vi "HFRR ADV v01.vi"() -> ()   [LabVIEW 2025] (continued)
          selector: w1771 -> [_ w1776]
          frame False {
          }
          frame True {
            n1472 = Not(x=w1776) -> (.not. x?=w1775:bool)
            n1473 = local write "CAMERA ROI MIN TEMP"(w1775) -> ()
            n1474 = call "IMAGE ANALYSIS.vi"("Enum"=POST_ANALYSIS_ENUM."MINIMIZE UI") -> ()  [unwired: 9 in, 2 out]
          }
        }
        n1475 = local write "CAMERA ROI MAX TEMP"(TRUE ("CAMERA ROI MIN TEMP")) -> ()
      }
      frame "Advance" {
        n1476 = local read "LIVE FEED MIN TEMP"() -> (w1782:bool)
        n1477 = local write "LIVE FEED MAX TEMP"(TRUE ("LIVE FEED MAX TEMP")) -> ()
        n1478 = local read "CAMERA ROI MIN TEMP"() -> (w1780:bool)
        n1479 = case shown="True" w1782 {
          selector: w1782 -> [_ w1789]
          frame False {
          }
          frame True {
            n1480 = Not(x=w1789) -> (.not. x?=w1788:bool)
            n1481 = local write "LIVE FEED MIN TEMP"(w1788) -> ()
            n1482 = call "CAMERA LIVE FEED FGV.vi"("Enum - Menu"=CAMERA_LIVE_FEED_ENUM."CAMERA MINIMIZE") -> ()  [unwired: 9 in, 2 out]
          }
        }
        n1483 = local write "CAMERA ROI MAX TEMP"(TRUE ("CAMERA ROI MAX TEMP")) -> ()
        n1484 = case shown="True" w1780 {
          selector: w1780 -> [_ w1786]
          frame False {
          }
          frame True {
            n1485 = Not(x=w1786) -> (.not. x?=w1785:bool)
            n1486 = local write "CAMERA ROI MIN TEMP"(w1785) -> ()
            n1487 = call "IMAGE ANALYSIS.vi"("Enum"=POST_ANALYSIS_ENUM."MINIMIZE UI") -> ()  [unwired: 9 in, 2 out]
          }
        }
      }
      frame "Mooha" {
        n1488 = local read "LIVE FEED MIN TEMP"() -> (w1792:bool)
        n1489 = local write "LIVE FEED MAX TEMP"(TRUE ("LIVE FEED MAX TEMP")) -> ()
        n1490 = local read "CAMERA ROI MIN TEMP"() -> (w1790:bool)
        n1491 = case shown="True" w1792 {
          selector: w1792 -> [_ w1799]
          frame False {
          }
          frame True {
            n1492 = Not(x=w1799) -> (.not. x?=w1798:bool)
            n1493 = local write "LIVE FEED MIN TEMP"(w1798) -> ()
            n1494 = call "CAMERA LIVE FEED FGV.vi"("Enum - Menu"=CAMERA_LIVE_FEED_ENUM."CAMERA MINIMIZE") -> ()  [unwired: 9 in, 2 out]
          }
        }
        n1495 = local write "CAMERA ROI MAX TEMP"(TRUE ("CAMERA ROI MAX TEMP")) -> ()
        n1496 = case shown="True" w1790 {
          selector: w1790 -> [_ w1796]
          frame False {
          }
          frame True {
            n1497 = Not(x=w1796) -> (.not. x?=w1795:bool)
            n1498 = local write "CAMERA ROI MIN TEMP"(w1795) -> ()
            n1499 = call "IMAGE ANALYSIS.vi"("Enum"=POST_ANALYSIS_ENUM."MINIMIZE UI") -> ()  [unwired: 9 in, 2 out]
          }
        }
      }
    }
    n1500 = local read "Auto Start Test"() -> (w1537:bool)
    n1501 = case shown="True" "sign in temp" {
      frame False {
      }
      frame True {
        w1572 = 1 ("y")
        n1502 = local read "USERNAME"() -> (w1578:string)
        n1503 = local read "USER ID"() -> (w1575:string)
        n1504 = call <vilib>:"Trim Whitespace.vi"("string"=w1578) -> ("trimmed string"=w1577:string)  [unwired: 1 in]
        n1505 = call <vilib>:"Trim Whitespace.vi"("string"=w1575) -> ("trimmed string"=w1576:string)  [unwired: 1 in]
        n1506 = String Length(string=w1577) -> (length=w1574:i32)
        n1507 = String Length(string=w1576) -> (length=w1573:i32)
        n1508 = Greater?(x=w1574, y=w1572) -> (0:w1571:bool)
        n1509 = Greater?(x=w1573, y=w1572) -> (0:w1570:bool)
        n1510 = And(x=w1571, y=w1570) -> (x .and. y?=w1569:bool)
        n1511 = case shown="True" w1569 {
          frame False {
            n1512 = property on="Sign In" class="Bool (strict)"("DisabledEnum"=T19."Disabled" ("Disabled")) -> ()  [unwired: 2 in, 2 out]
          }
          frame True {
            n1513 = property on="Sign In" class="Bool (strict)"("DisabledEnum"=T19."Enabled" ("Disabled")) -> ()  [unwired: 2 in, 2 out]
          }
        }
      }
    }
    n1514 = local read "Air Temperature"() -> (w1554:bool)
    n1515 = local read "Coefficient Of Friction"() -> (w1555:bool)
    n1516 = case shown="False" w1537 {
      frame False {
        n1517 = local read "Auto stop temp"() -> (w1566:bool)
        n1518 = case shown="True" w1566 {
          frame False {
          }
          frame True {
            n1519 = local write "Auto Start Temp"(FALSE ("Auto Start Temp")) -> ()
          }
        }
      }
      frame True {
        "Auto stop temp" <- TRUE ("Auto stop temp")
      }
    }
    n1520 = local read "Humidity 3"() -> (w1553:bool)
    n1521 = case shown="\"HOME\"" w1563 {
      frame "HOME" {
        n1522 = local write "main tab sub"(enum32{"Page 1", "Page 2"}."Page 1" ("main tab sub")) -> ()
      }
      frame Default {
        n1523 = local write "main tab sub"(enum32{"Page 1", "Page 2"}."Page 2" ("main tab sub")) -> ()
      }
    }
    n1524 = case shown="True" w1562 {
      selector: w1562 -> [_ w1914]
      frame False {
      }
      frame True {
        n1525 = Not(x=w1914) -> (.not. x?=w1913:bool)
        n1526 = local write "Sign In"(w1913) -> ()
        n1527 = local write "Main Dashboard Buttons"(T25."Test Setup" ("Main Dashboard Buttons")) -> ()
      }
    }
    n1528 = case shown="\"Numeric Display\", Default" "Num/Graph" {
      frame "Numeric Display", Default {
        n1529 = property on="Single/Multiple" class="RadioBtnsControl (strict)"("Visible"=FALSE) -> ()  [unwired: 2 in, 2 out]
        n1530 = property on="Single - Graph" class="Ring (strict)"("Visible"=FALSE) -> ()  [unwired: 2 in, 2 out]
        n1531 = local write "Main Tab Display"(T6."Dashboard 1" ("Main Tab Display")) -> ()
      }
      frame "Graph Display" {
        n1532 = property on="Single/Multiple" class="RadioBtnsControl (strict)"("Visible"=TRUE) -> ()  [unwired: 2 in, 2 out]
        n1533 = case shown="\"Multiple\"" "Single/Multiple" {
          frame "Single ", Default {
            n1534 = property on="Single - Graph" class="Ring (strict)"("Visible"=TRUE) -> ()  [unwired: 2 in, 2 out]
            n1535 = local write "Main Tab Display"(T6."Dashboard 3" ("Main Tab Display")) -> ()
          }
          frame "Multiple" {
            n1536 = property on="Single - Graph" class="Ring (strict)"("Visible"=FALSE) -> ()  [unwired: 2 in, 2 out]
            n1537 = local write "Main Tab Display"(T6."Dashboard 2" ("Main Tab Display")) -> ()
          }
        }
      }
    }
    n1538 = local read "Stroke"() -> (w1552:bool)
    n1539 = local read "USERNAME"() -> (w1557:string)
    n1540 = case shown="True" w1555 {
      selector: w1555 -> [_ w1839]
      frame False {
      }
      frame True {
        n1541 = Not(x=w1839) -> (.not. x?=w1838:bool)
        n1542 = local write "Coefficient Of Friction"(w1838) -> ()
        n1543 = local write "Tab Control 2"(T8."Coefficient Of Friction" ("Tab Control 2")) -> ()
      }
    }
    n1544 = case shown="True" w1554 {
      selector: w1554 -> [_ w1836]
      frame False {
      }
      frame True {
        n1545 = Not(x=w1836) -> (.not. x?=w1834:bool)
        n1546 = local write "Air Temperature"(w1834) -> ()
        n1547 = local write "Tab Control 2"(T8."Air Temperature" ("Tab Control 2")) -> ()
      }
    }
    n1548 = case shown="True" w1552 {
      selector: w1552 -> [_ w1830]
      frame False {
      }
      frame True {
        n1549 = Not(x=w1830) -> (.not. x?=w1828:bool)
        n1550 = local write "Stroke"(w1828) -> ()
        n1551 = local write "Tab Control 2"(T8."Stroke" ("Tab Control 2")) -> ()
      }
    }
    n1552 = local write "tested by"(w1557) -> ()
    n1553 = case shown="True" w1553 {
      selector: w1553 -> [_ w1833]
      frame False {
      }
      frame True {
        n1554 = Not(x=w1833) -> (.not. x?=w1831:bool)
        n1555 = local write "Humidity 3"(w1831) -> ()
        n1556 = local write "Tab Control 2"(T8."Humidity" ("Tab Control 2")) -> ()
      }
    }
    n1557 = case shown="\"Calibration\"" "Main Dashboard Buttons" {
      tunnel: [T4."HOME" ("Main Tab") T4."Test Setup" ("Main Tab") T4."Acquire" ("Main Tab") T4."Adv Scar" ("Main Tab") T4."Adv Scar Report" ("Main Tab") T4."Compare Files" ("Main Tab") T4."Calibration" ("Main Tab") T4."About" ("Main Tab") T4."Advance" ("Main Tab")] -> w1536
      frame "Home", Default {
      }
      frame "Test Setup" {
      }
      frame "Dashboard" {
      }
      frame "Imaging" {
      }
      frame "Report" {
      }
      frame "Analysis" {
      }
      frame "Calibration" {
      }
      frame "About" {
      }
      frame "Advance" {
      }
    }
    n1558 = Wait (ms)(milliseconds to wait=u32 100) -> ()  [unwired: 1 out]
    n1559 = local read "Main Tab Display"() -> (w1556:T6)
    n1560 = local write "Main Tab"(w1536) -> ()
    n1561 = case shown="\"Dashboard 3\"" w1556 {
      frame "Dashboard 1", Default {
        n1562 = property on="Reset Graph" class="Bool (strict)"("Visible"=FALSE) -> ()  [unwired: 2 in, 2 out]
      }
      frame "Dashboard 2" {
        n1563 = property on="Reset Graph" class="Bool (strict)"("Visible"=TRUE) -> ()  [unwired: 2 in, 2 out]
      }
      frame "Dashboard 3" {
        n1564 = property on="Reset Graph" class="Bool (strict)"("Visible"=TRUE) -> ()  [unwired: 2 in, 2 out]
      }
    }
    n1565 = local read "SCAR MEASURMENT"() -> (w1544:enum32{"Auto Scar", "Manual Scar"})
    n1566 = local read "Humidity"() -> (w1558:bool)
    n1567 = local read "Cap Live Image"() -> (w1541:bool)
    n1568 = local read "Sample Temperature"() -> (w1551:bool)
    n1569 = local read "Air Temp vs Humidity"() -> (w1549:bool)
    n1570 = local read "Frequency"() -> (w1550:bool)
    n1571 = case shown="False" w1558 {
      frame False {
        n1572 = local write "Humidity On Command"(TRUE ("Humidity On Command")) -> ()
        n1573 = case shown="True" "Humidity Off Command" {
          selector: "Humidity Off Command" -> [_ w1846]
          frame False {
          }
          frame True {
            n1574 = stacked-sequence {
              frame #0 {
                n1575 = local read "WriteHumidity"() -> (w1848:string[])
                n1576 = Insert Into Array(array=w1848, new element="R;1" ("new element/subarray")) -> (w1847:string[])  [unwired: 1 in]
                n1577 = local write "WriteHumidity"(w1847) -> ()
              }
              frame #1 {
                n1578 = Wait (ms)(milliseconds to wait=u32 500) -> ()  [unwired: 1 out]
              }
              frame #2 {
                n1579 = local read "WriteHumidity"() -> (w1852:string[])
                n1580 = local read "EVENT LOG"() -> (w1856:string)
                n1581 = call "Event Log.vi"("Content"="Humidity Control Off" ("string"), "EVENT LOG"=w1856) -> ("EVENT LOG"=w1857:string)  [unwired: 8 in, 1 out]
                n1582 = local write "EVENT LOG"(w1857) -> ()
                n1583 = Insert Into Array(array=w1852, new element="R;1" ("new element/subarray")) -> (w1853:string[])  [unwired: 1 in]
                n1584 = local write "WriteHumidity"(w1853) -> ()
                n1585 = local write "Humidity 2"(TRUE ("Humidity")) -> ()
              }
            }
            n1586 = Not(x=w1846) -> (.not. x?=w1845:bool)
            n1587 = local write "Humidity Off Command"(w1845) -> ()
          }
        }
      }
      frame True {
        n1588 = local write "Humidity Off Command"(TRUE ("Humidity Off Command")) -> ()
        n1589 = case shown="False" "Humidity On Command" {
          selector: "Humidity On Command" -> [_ w1861]
          frame False {
          }
          frame True {
            n1590 = stacked-sequence {
              frame #0 {
                n1591 = local read "Set Rh"() -> (w1867:dbl)
                n1592 = local read "WriteHumidity"() -> (w1863:string[])
                n1593 = Number To Fractional String(number=w1867, precision (6)=i16 2) -> (F-format string=w1868:string)  [unwired: 2 in]
                n1594 = Concatenate Strings("M;" ("new element/subarray"), w1868) -> (w1866:string)
                n1595 = Insert Into Array(array=w1863, new element=w1866) -> (w1862:string[])  [unwired: 1 in]
                n1596 = local write "WriteHumidity"(w1862) -> ()
              }
              frame #1 {
                n1597 = Wait (ms)(milliseconds to wait=u32 500) -> ()  [unwired: 1 out]
              }
              frame #2 {
                n1598 = local read "WriteHumidity"() -> (w1871:string[])
                n1599 = local read "Set Rh"() -> (w1875:dbl)
                n1600 = Number To Fractional String(number=w1875, precision (6)=i16 2) -> (F-format string=w1876:string)  [unwired: 2 in]
                n1601 = Concatenate Strings("M;" ("new element/subarray"), w1876) -> (w1874:string)
                n1602 = Insert Into Array(array=w1871, new element=w1874) -> (w1870:string[])  [unwired: 1 in]
                n1603 = local write "WriteHumidity"(w1870) -> ()
              }
              frame #3 {
                n1604 = Wait (ms)(milliseconds to wait=u32 500) -> ()  [unwired: 1 out]
              }
              frame #4 {
                (unwired) "% RH" ("string")
                (unwired) i16 2 ("precision (6)")
                (unwired) "M;" ("new element/subarray")
                n1605 = local read "Set Rh"() -> (w1885:dbl)
                n1606 = local read "WriteHumidity"() -> (w1878:string[])
                n1607 = Number To Fractional String(number=w1885, precision (6)=i16 2) -> (F-format string=w1882:string)  [unwired: 2 in]
                n1608 = Concatenate Strings("M;" ("new element/subarray"), w1882) -> (w1886:string)
                n1609 = Concatenate Strings("Humidity Set to : " ("string"), w1882, "% RH" ("string")) -> (w1880:string)
                n1610 = Insert Into Array(array=w1878, new element=w1886) -> (w1879:string[])  [unwired: 1 in]
                n1611 = disable-structure shown="Enabled" {
                  frame Enabled {
                    n1612 = local read "EVENT LOG"() -> (w1889:string)
                    n1613 = call "Event Log.vi"("Content"="Humidity Control On", "EVENT LOG"=w1889) -> ("EVENT LOG"=w1890:string)  [unwired: 8 in, 1 out]
                    n1614 = local write "EVENT LOG"(w1890) -> ()
                  }
                  frame Disabled {
                  }
                }
                n1615 = disable-structure shown="Enabled" {
                  disable-tunnel: w1880 -> [_ _]
                  frame Enabled {
                    n1616 = local read "EVENT LOG"() -> (w1892:string)
                    n1617 = call "Event Log.vi"("Content"="Humidity Control On", "EVENT LOG"=w1892) -> ("EVENT LOG"=w1893:string)  [unwired: 8 in, 1 out]
                    n1618 = local write "EVENT LOG"(w1893) -> ()
                  }
                  frame Disabled {
                  }
                }
                n1619 = local write "WriteHumidity"(w1879) -> ()
              }
            }
            n1620 = Not(x=w1861) -> (.not. x?=w1860:bool)
            n1621 = local write "Humidity On Command"(w1860) -> ()
          }
        }
      }
    }
    n1622 = Equal?(x=w1544, y=enum32{"Auto Scar", "Manual Scar"}."Auto Scar" ("SCAR MEASURMENT")) -> (x = y?=w1540:bool)
    n1623 = local read "TEST STANDARD"() -> (w1547:T5)
    n1624 = And(x=w1541, y=w1540) -> (x .and. y?=w1542:bool)
    n1625 = case shown="True" w1542 {
      selector: w1542 -> [_ w1645]
      tunnel: errorcluster {"status"=FALSE, "code"=0, "source"=""} ("error in (no error) 3") -> [_ w1646]
      frame False {
      }
      frame True {
        n1626 = stacked-sequence {
          tunnel: w1646 -> [_ _ _ _ _ _ _ w1694]
          tunnel: w1645 -> [_ _ _ _ _ w1675 _ _]
          frame #0 {
            n1627 = call "CAMERA LIVE FEED FGV.vi"("Enum - Menu"=CAMERA_LIVE_FEED_ENUM."CAMERA MINIMIZE") -> ()  [unwired: 9 in, 2 out]
          }
          frame #1 {
            n1628 = property on="Auto Scar Check  2" class="Clust (strict)"("Visible"=TRUE) -> ()  [unwired: 2 in, 2 out]
          }
          frame #2 {
            n1629 = String To Path(string="C:\\LAB-IQ\\Image Calibrate v01.dcf") -> (path=w1651:path)
            n1630 = Open/Create/Replace File ("Open File")(file path (use dialog)=w1651) -> (refnum out=w1652:refnum<file>)  [unwired: 5 in, 2 out]
            n1631 = for {
              N: 4 -> [_]
              tunnel: w1652 -> [w1658]
              i -> [w1654]
              n1632 = Read from Text File ("Read File")(file (use dialog)=w1658) -> (text=w1659:string)  [unwired: 3 in, 3 out]
              n1633 = String Subset(string=w1659, offset (0)=6, length (rest)=10 ("length (rest)")) -> (substring=w1655:string)
              n1634 = Fract/Exp String To Number(string=w1655) -> (number=w1653:dbl)  [unwired: 3 in, 1 out]
              n1635 = case shown="0" w1654 {
                tunnel: w1653 -> [w1660 w1661 _ w1662 _]
                frame 0 {
                  "5x Gain" <- w1660
                }
                frame 1 {
                  "10x Gain" <- w1661
                }
                frame 2 {
                }
                frame 3 {
                  "100x gain" <- w1662
                }
                frame 4, Default {
                }
              }
            }
          }
          frame #3 {
            n1636 = local read "FILE 3"() -> (w1668:string)
            n1637 = call <vilib>:"Trim Whitespace.vi"("string"="C:\\LAB-IQ\\images\\") -> ("trimmed string"=w1670:string)  [unwired: 1 in]
            n1638 = String To Path(string=w1670) -> (path=w1669:path)
            n1639 = Concatenate Strings(w1668, ".png" ("string")) -> (w1667:string)
            n1640 = Build Path(base path=w1669, name or relative path=w1667) -> (appended path=w1665:path)
            "Image path" <- w1665
            n1641 = Path To String(path=w1665) -> (string=w1664:string)
            n1642 = call "CAMERA LIVE FEED FGV.vi"("Enum - Menu"=CAMERA_LIVE_FEED_ENUM."CAMERA SAVE", "Image Path"=w1664) -> ()  [unwired: 8 in, 2 out]
          }
          frame #4 {
            n1643 = One Button Dialog(message="Image saved successfully") -> ()  [unwired: 1 in, 1 out]
          }
          frame #5 {
            n1644 = local read "TEST STANDARD"() -> (w1674:T5)
            n1645 = local read "Magnification len live scar"() -> (w1686:string)
            n1646 = Not(x=w1675) -> (.not. x?=w1676:bool)
            n1647 = local write "Cap Live Image"(w1676) -> ()
            n1648 = case shown="\"ISO 12156\"" w1674 {
              tunnel: ["ASTM D6079" "ISO 12156"] -> w1673
              frame "ASTM D6079", Default {
              }
              frame "ISO 12156" {
              }
            }
            n1649 = case shown="\"5x\", Default" w1686 {
              tunnel: [w1689 w1690] -> w1685
              frame "5x", Default {
                n1650 = local read "5x Gain"() -> (w1689:dbl)
              }
              frame "10x" {
                # "5x"
                n1651 = local read "10x Gain"() -> (w1690:dbl)
              }
            }
            n1652 = local read "Image path"() -> (w1684:path)
            n1653 = local read "FILE 3"() -> (w1677:string)
            n1654 = call "EDGE DETCTION.vi"("GAIN VALUE"=w1685, "Image Path"=w1684) -> ("error out"=w1683:errorcluster, "return value"=w1682:cluster{string, string, dbl, dbl, dbl})  [unwired: 8 in]
            n1655 = Bundle By Name(cluster=T26 {"File Name"="", "Test Method"="", "Operator"="", "Fuel Description"="", "Date and time"=""} ("Main Ref"), "File Name"=w1677, "Test Method"=w1673) -> (w1678:T26)
            n1656 = call "duf file read.vi"("error in (no error)"=w1683, "Main Ref"=w1678) -> ("error out"=w1681:errorcluster, "Main Ref 2"=w1679:T26)  [unwired: 8 in]
            n1657 = call "EDGE DETECTION REPORT.vi"("error in (no error)"=w1681, "return value 2"=w1682, "Main Ref"=w1679) -> ()  [unwired: 8 in, 1 out]
          }
          frame #6 {
            n1658 = property on="Auto Scar Check  2" class="Clust (strict)"("Visible"=FALSE) -> ()  [unwired: 2 in, 2 out]
          }
          frame #7 {
            n1659 = call "CAMERA LIVE FEED FGV.vi"("Enum - Menu"=CAMERA_LIVE_FEED_ENUM."CAMERA MINIMIZE", "error in (no error)"=w1694) -> ()  [unwired: 8 in, 2 out]
            n1660 = local write "Main Dashboard Buttons"(T1."Home" ("Main Dashboard Buttons")) -> ()
            n1661 = local write "Main Tab"(T4."HOME" ("Main Tab")) -> ()
          }
        }
      }
    }
    n1662 = local read "Heater Button"() -> (w1548:bool)
    n1663 = case shown="True" w1550 {
      selector: w1550 -> [_ w1824]
      frame False {
      }
      frame True {
        n1664 = Not(x=w1824) -> (.not. x?=w1822:bool)
        n1665 = local write "Frequency"(w1822) -> ()
        n1666 = local write "Tab Control 2"(T8."Frequency" ("Tab Control 2")) -> ()
      }
    }
    n1667 = case shown="True" w1549 {
      selector: w1549 -> [_ w1821]
      frame False {
      }
      frame True {
        n1668 = Not(x=w1821) -> (.not. x?=w1819:bool)
        n1669 = local write "Air Temp vs Humidity"(w1819) -> ()
        n1670 = local write "Tab Control 2"(T8."Air Temp vs Rh" ("Tab Control 2")) -> ()
      }
    }
    n1671 = case shown="True" w1551 {
      selector: w1551 -> [_ w1827]
      frame False {
      }
      frame True {
        n1672 = Not(x=w1827) -> (.not. x?=w1825:bool)
        n1673 = local write "Sample Temperature"(w1825) -> ()
        n1674 = local write "Tab Control 2"(T8."Sample Temperature" ("Tab Control 2")) -> ()
      }
    }
    n1675 = case shown="\"Custom\"" w1547 {
      frame "ASTM D6079", Default {
        w1800 = "ASTM D6079 TEST CONDITIONS" ("Standard 2")
        n1676 = local write "Standard 2"(w1800) -> ()
        n1677 = local write "Standard"(w1800) -> ()
      }
      frame "ISO 12156" {
        w1801 = "ISO 12156 TEST CONDITIONS" ("Standard 2")
        n1678 = local write "Standard 2"(w1801) -> ()
        n1679 = local write "Standard"(w1801) -> ()
      }
      frame "CEC F-096-A-06" {
        w1802 = "CEC F-096-A-06 TEST CONDITIONS" ("Standard 2")
        n1680 = local write "Standard 2"(w1802) -> ()
        n1681 = local write "Standard"(w1802) -> ()
      }
      frame "Custom" {
        w1803 = "CUSTOM TEST CONDITIONS" ("Standard 2")
        n1682 = local write "Standard 2"(w1803) -> ()
        n1683 = local write "Standard"(w1803) -> ()
      }
    }
    n1684 = case shown="True" w1548 {
      frame False {
        n1685 = local write "Temperature On Command"(TRUE ("Temperature On Command")) -> ()
        n1686 = case shown="True" "Temperature Off Command" {
          selector: "Temperature Off Command" -> [_ w1807]
          frame False {
          }
          frame True {
            n1687 = Not(x=w1807) -> (.not. x?=w1806:bool)
            n1688 = local read "EVENT LOG"() -> (w1810:string)
            n1689 = local write "Temperature Off Command"(w1806) -> ()
            n1690 = call "Event Log.vi"("Content"="Heater Off", "EVENT LOG"=w1810) -> ("EVENT LOG"=w1809:string)  [unwired: 8 in, 1 out]
            n1691 = local write "EVENT LOG"(w1809) -> ()
          }
        }
      }
      frame True {
        n1692 = local write "Temperature Off Command"(TRUE ("Temperature Off Command")) -> ()
        n1693 = case shown="True" "Temperature On Command" {
          selector: "Temperature On Command" -> [_ w1814]
          frame False {
          }
          frame True {
            n1694 = Not(x=w1814) -> (.not. x?=w1813:bool)
            n1695 = local write "Temperature On Command"(w1813) -> ()
            n1696 = disable-structure shown="Enabled" {
              disable-tunnel: "Heater On" -> [w1816 _]
              frame Enabled {
                n1697 = local read "EVENT LOG"() -> (w1817:string)
                n1698 = call "Event Log.vi"("Content"=w1816, "EVENT LOG"=w1817) -> ("EVENT LOG"=w1818:string)  [unwired: 8 in, 1 out]
                n1699 = local write "EVENT LOG"(w1818) -> ()
              }
              frame Disabled {
              }
            }
          }
        }
      }
    }
    n1700 = local read "Main Tab"() -> (w1539:T4)
    n1701 = case shown="\"About\"" w1539 {
      frame "HOME", Default {
        w1581 = T19."Enabled" ("Disabled")
        n1702 = local read "Service Password enable"() -> (w1583:bool)
        n1703 = property on="Imaging" class="Bool (strict)"("DisabledEnum"=w1581) -> ()  [unwired: 2 in, 2 out]
        n1704 = property on="Dashboard" class="Bool (strict)"("DisabledEnum"=w1581) -> ()  [unwired: 2 in, 2 out]
        n1705 = property on="Test Setup" class="Bool (strict)"("DisabledEnum"=w1581) -> ()  [unwired: 2 in, 2 out]
        n1706 = property on="Analysis" class="Bool (strict)"("DisabledEnum"=w1581) -> ()  [unwired: 2 in, 2 out]
        n1707 = property on="Home" class="Bool (strict)"("DisabledEnum"=w1581) -> ()  [unwired: 2 in, 2 out]
        n1708 = property on="Report" class="Bool (strict)"("DisabledEnum"=w1581) -> ()  [unwired: 2 in, 2 out]
        n1709 = property on="Main Dashboard Buttons" class="RadioBtnsControl (strict)"("DisabledEnum"=w1581) -> ()  [unwired: 2 in, 2 out]
        n1710 = property on="Calibration" class="Bool (strict)"("DisabledEnum"=w1581) -> ()  [unwired: 2 in, 2 out]
        n1711 = case shown="True" w1583 {
          tunnel: [T19."Disabled" ("Disabled") T19."Enabled" ("Disabled")] -> w1582
          frame False {
          }
          frame True {
          }
        }
        n1712 = property on="About" class="Bool (strict)"("DisabledEnum"=w1582) -> ()  [unwired: 2 in, 2 out]
      }
      frame "Test Setup" {
        w1588 = T19."Enabled" ("Disabled")
        n1713 = local read "Service Password enable"() -> (w1587:bool)
        n1714 = property on="Dashboard" class="Bool (strict)"("DisabledEnum"=T19."Disabled" ("Disabled")) -> ()  [unwired: 2 in, 2 out]
        n1715 = property on="Imaging" class="Bool (strict)"("DisabledEnum"=w1588) -> ()  [unwired: 2 in, 2 out]
        n1716 = property on="Analysis" class="Bool (strict)"("DisabledEnum"=w1588) -> ()  [unwired: 2 in, 2 out]
        n1717 = property on="Home" class="Bool (strict)"("DisabledEnum"=w1588) -> ()  [unwired: 2 in, 2 out]
        n1718 = property on="Report" class="Bool (strict)"("DisabledEnum"=w1588) -> ()  [unwired: 2 in, 2 out]
        n1719 = property on="Test Setup" class="Bool (strict)"("DisabledEnum"=w1588) -> ()  [unwired: 2 in, 2 out]
        n1720 = case shown="True" w1587 {
          tunnel: [T19."Disabled" ("Disabled") T19."Enabled" ("Disabled")] -> w1586
          frame False {
          }
          frame True {
          }
        }
        n1721 = property on="About" class="Bool (strict)"("DisabledEnum"=w1586) -> ()  [unwired: 2 in, 2 out]
      }
      frame "Adv Scar" {
        w1595 = T19."Enabled" ("Disabled")
        n1722 = property on="Dashboard" class="Bool (strict)"("DisabledEnum"=T19."Disabled" ("Disabled")) -> ()  [unwired: 2 in, 2 out]
        n1723 = property on="Imaging" class="Bool (strict)"("DisabledEnum"=w1595) -> ()  [unwired: 2 in, 2 out]
        n1724 = property on="Analysis" class="Bool (strict)"("DisabledEnum"=w1595) -> ()  [unwired: 2 in, 2 out]
        n1725 = property on="Home" class="Bool (strict)"("DisabledEnum"=w1595) -> ()  [unwired: 2 in, 2 out]
        n1726 = property on="Report" class="Bool (strict)"("DisabledEnum"=w1595) -> ()  [unwired: 2 in, 2 out]
        n1727 = property on="Test Setup" class="Bool (strict)"("DisabledEnum"=w1595) -> ()  [unwired: 2 in, 2 out]
        n1728 = local read "Service Password enable"() -> (w1593:bool)
        n1729 = case shown="True" w1593 {
          tunnel: [T19."Disabled" ("Disabled") T19."Enabled" ("Disabled")] -> w1592
          frame False {
          }
          frame True {
          }
        }
        n1730 = property on="About" class="Bool (strict)"("DisabledEnum"=w1592) -> ()  [unwired: 2 in, 2 out]
      }
      frame "Calibration" {
        w1598 = T19."Enabled" ("Disabled")
        n1731 = property on="Dashboard" class="Bool (strict)"("DisabledEnum"=T19."Disabled" ("Disabled")) -> ()  [unwired: 2 in, 2 out]
        n1732 = property on="Imaging" class="Bool (strict)"("DisabledEnum"=w1598) -> ()  [unwired: 2 in, 2 out]
        n1733 = property on="Analysis" class="Bool (strict)"("DisabledEnum"=w1598) -> ()  [unwired: 2 in, 2 out]
        n1734 = property on="Home" class="Bool (strict)"("DisabledEnum"=w1598) -> ()  [unwired: 2 in, 2 out]
        n1735 = property on="Report" class="Bool (strict)"("DisabledEnum"=w1598) -> ()  [unwired: 2 in, 2 out]
        n1736 = property on="Test Setup" class="Bool (strict)"("DisabledEnum"=w1598) -> ()  [unwired: 2 in, 2 out]
        n1737 = local read "Service Password enable"() -> (w1600:bool)
        n1738 = property on="Calibration" class="Bool (strict)"("DisabledEnum"=w1598) -> ()  [unwired: 2 in, 2 out]
        n1739 = case shown="True" w1600 {
          tunnel: [T19."Disabled" ("Disabled") T19."Enabled" ("Disabled")] -> w1599
          frame False {
          }
          frame True {
          }
        }
        n1740 = property on="About" class="Bool (strict)"("DisabledEnum"=w1599) -> ()  [unwired: 2 in, 2 out]
      }
      frame "Adv Scar Report" {
        w1606 = T19."Enabled" ("Disabled")
        n1741 = property on="Dashboard" class="Bool (strict)"("DisabledEnum"=T19."Disabled" ("Disabled")) -> ()  [unwired: 2 in, 2 out]
        n1742 = property on="Imaging" class="Bool (strict)"("DisabledEnum"=w1606) -> ()  [unwired: 2 in, 2 out]
        n1743 = property on="Analysis" class="Bool (strict)"("DisabledEnum"=w1606) -> ()  [unwired: 2 in, 2 out]
        n1744 = property on="Home" class="Bool (strict)"("DisabledEnum"=w1606) -> ()  [unwired: 2 in, 2 out]
        n1745 = property on="Report" class="Bool (strict)"("DisabledEnum"=w1606) -> ()  [unwired: 2 in, 2 out]
        n1746 = property on="Test Setup" class="Bool (strict)"("DisabledEnum"=w1606) -> ()  [unwired: 2 in, 2 out]
        n1747 = local read "Service Password enable"() -> (w1605:bool)
        n1748 = case shown="True" w1605 {
          tunnel: [T19."Disabled" ("Disabled") T19."Enabled" ("Disabled")] -> w1604
          frame False {
          }
          frame True {
          }
        }
        n1749 = property on="About" class="Bool (strict)"("DisabledEnum"=w1604) -> ()  [unwired: 2 in, 2 out]
      }
      frame "Compare Files" {
        w1612 = T19."Enabled" ("Disabled")
        n1750 = local read "Service Password enable"() -> (w1611:bool)
        n1751 = property on="Dashboard" class="Bool (strict)"("DisabledEnum"=T19."Disabled" ("Disabled")) -> ()  [unwired: 2 in, 2 out]
        n1752 = property on="Imaging" class="Bool (strict)"("DisabledEnum"=w1612) -> ()  [unwired: 2 in, 2 out]
        n1753 = property on="Analysis" class="Bool (strict)"("DisabledEnum"=w1612) -> ()  [unwired: 2 in, 2 out]
        n1754 = property on="Home" class="Bool (strict)"("DisabledEnum"=w1612) -> ()  [unwired: 2 in, 2 out]
        n1755 = property on="Report" class="Bool (strict)"("DisabledEnum"=w1612) -> ()  [unwired: 2 in, 2 out]
        n1756 = property on="Test Setup" class="Bool (strict)"("DisabledEnum"=w1612) -> ()  [unwired: 2 in, 2 out]
        n1757 = case shown="True" w1611 {
          tunnel: [T19."Disabled" ("Disabled") T19."Enabled" ("Disabled")] -> w1610
          frame False {
          }
          frame True {
          }
        }
        n1758 = property on="About" class="Bool (strict)"("DisabledEnum"=w1610) -> ()  [unwired: 2 in, 2 out]
      }
      frame "Acquire" {
        n1759 = local read "Service Password enable"() -> (w1617:bool)
        n1760 = property on="Test Setup" class="Bool (strict)"("DisabledEnum"=T19."Disabled" ("Disabled")) -> ()  [unwired: 2 in, 2 out]
        n1761 = local read "Auto Start Test"() -> (w1619:bool)
        n1762 = local read "RUN"() -> (w1621:bool)
        n1763 = case shown="True" w1617 {
          tunnel: [T19."Disabled" ("Disabled") T19."Enabled" ("Disabled")] -> w1618
          frame False {
          }
          frame True {
          }
        }
        n1764 = Or(x=w1621, y=w1619) -> (x .or. y?=w1620:bool)
        n1765 = case shown="True" w1620 {
          tunnel: [T19."Enabled" ("Disabled") T19."Disabled" ("Disabled")] -> w1616
          frame False {
          }
          frame True {
          }
        }
        n1766 = property on="About" class="Bool (strict)"("DisabledEnum"=w1618) -> ()  [unwired: 2 in, 2 out]
        n1767 = property on="Imaging" class="Bool (strict)"("DisabledEnum"=w1616) -> ()  [unwired: 2 in, 2 out]
        n1768 = property on="Dashboard" class="Bool (strict)"("DisabledEnum"=w1616) -> ()  [unwired: 2 in, 2 out]
        n1769 = property on="Analysis" class="Bool (strict)"("DisabledEnum"=w1616) -> ()  [unwired: 2 in, 2 out]
        n1770 = property on="Home" class="Bool (strict)"("DisabledEnum"=w1616) -> ()  [unwired: 2 in, 2 out]
        n1771 = property on="Report" class="Bool (strict)"("DisabledEnum"=w1616) -> ()  [unwired: 2 in, 2 out]
        n1772 = property on="Calibration" class="Bool (strict)"("DisabledEnum"=w1616) -> ()  [unwired: 2 in, 2 out]
      }
      frame "About" {
        n1773 = local read "FILE"() -> (w1635:string)
        n1774 = local read "TEST FILE NAM,E SAVED"() -> (w1628:bool)
        n1775 = call <vilib>:"Trim Whitespace.vi"("string"=w1635) -> ("trimmed string"=w1634:string)  [unwired: 1 in]
        n1776 = local read "Auto Start Test"() -> (w1638:bool)
        n1777 = String Length(string=w1634) -> (length=w1633:i32)
        n1778 = Greater?(x=w1633, y=1) -> (0:w1630:bool)
        n1779 = And(x=w1630, y=w1628) -> (x .and. y?=w1629:bool)
        n1780 = local read "RUN"() -> (w1640:bool)
        n1781 = case shown="True" w1629 {
          tunnel: [T19."Disabled" ("Disabled") T19."Enabled" ("Disabled")] -> w1631
          frame False {
          }
          frame True {
          }
        }
        n1782 = Or(x=w1640, y=w1638) -> (x .or. y?=w1639:bool)
        n1783 = property on="About" class="Bool (strict)"("DisabledEnum"=T19."Enabled" ("Disabled")) -> ()  [unwired: 2 in, 2 out]
        n1784 = case shown="False" w1639 {
          tunnel: [T19."Enabled" ("Disabled") T19."Disabled" ("Disabled")] -> w1637
          frame False {
          }
          frame True {
          }
        }
        n1785 = property on="Dashboard" class="Bool (strict)"("DisabledEnum"=w1631) -> ()  [unwired: 2 in, 2 out]
        n1786 = property on="Test Setup" class="Bool (strict)"("DisabledEnum"=T19."Disabled" ("Disabled")) -> ()  [unwired: 2 in, 2 out]
        n1787 = property on="Imaging" class="Bool (strict)"("DisabledEnum"=w1637) -> ()  [unwired: 2 in, 2 out]
        n1788 = property on="Analysis" class="Bool (strict)"("DisabledEnum"=w1637) -> ()  [unwired: 2 in, 2 out]
        n1789 = property on="Home" class="Bool (strict)"("DisabledEnum"=w1637) -> ()  [unwired: 2 in, 2 out]
        n1790 = property on="Report" class="Bool (strict)"("DisabledEnum"=w1637) -> ()  [unwired: 2 in, 2 out]
      }
    }
    n1791 = local read "Quit"() -> (w1565:bool)
    "Single" <- "Single - Graph"
  }
  n1792 = disable-structure shown="Disabled" {
    disable-tunnel: [w1918 _] -> w47
    disable-tunnel: _ -> [w1917 _]
    frame Disabled {
      n1793 = while {
        tunnel: w1917 -> [_]
        tunnel: [w1919] -> w1918
        tunnel: [w1920] -> _
        i -> [w1920]
        stop <- w1919 stop-if-true
        w1936 = u16 10 items=["1.0"=10, "1.5"=15, "2.0"=20] ("stop bits (10: 1 bit)")
        n1794 = Wait (ms)(milliseconds to wait=u32 10) -> ()  [unwired: 1 out]
        n1795 = call-poly "VISA Configure Serial Port"("VISA resource name"=refnum<visa-resource-name> "ASRL1::INSTR" ("COM PORT"), "timeout (10sec)"=u32 10, "baud rate (9600)"=u32 57600, "data bits (8)"=u16 8, "stop bits (10: 1 bit)"=w1936) -> ("VISA resource name out"=w1922:refnum<visa-resource-name>, "error out"=w1931:errorcluster)  [unwired: 9 in]
        n1796 = VISA Read(VISA resource name=w1922, byte count=u32 2 ("byte count (0)")) -> (read buffer=w1930:string)  [unwired: 1 in, 3 out]
        n1797 = String Subset(string=w1930, offset (0)=0, length (rest)=2 ("length (rest)")) -> (substring=w1929:string)
        n1798 = Match Pattern(string=w1929, regular expression="<>") -> (offset past match=w1926:i32)  [unwired: 1 in, 3 out]
        n1799 = Greater Or Equal?(x=w1926, y=0) -> (x >= y?=w1921:bool)
        n1800 = case shown="True" w1921 {
          tunnel: w1922 -> [_ w1940]
          tunnel: w1931 -> [_ w1939]
          frame False {
          }
          frame True {
            n1801 = VISA Read(VISA resource name=w1940, byte count=u32 32 ("byte count (0)"), error in (no error)=w1939) -> (read buffer=w1938:string)  [unwired: 3 out]
            n1802 = String Subset(string=w1938, offset (0)=0, length (rest)=8 ("length (rest)")) -> (substring=w1942:string)
            n1803 = String Subset(string=w1938, offset (0)=8, length (rest)=8 ("length (rest)")) -> (substring=w1943:string)
            n1804 = Decimal String To Number(string=w1943) -> (number=w1950:i32)  [unwired: 2 in, 1 out]
            n1805 = Decimal String To Number(string=w1942) -> (number=w1946:i32)  [unwired: 2 in, 1 out]
            n1806 = Divide(x=w1950, y=10000) -> ()  [unwired: 1 out]
            n1807 = Divide(x=w1946, y=1000000) -> ()  [unwired: 1 out]
          }
        }
        n1808 = local read "Quit"() -> (w1919:bool)
      }
    }
    frame Enabled {
    }
  }
  n1809 = Tick Count (ms)() -> (millisecond timer value=w9:u32)
  n1810 = while {
    shift-right: [w1996] -> _
    shift-left: w11 -> [w2000]
    shift-right: [w1995] -> _
    shift-left: w10 -> [w1999]
    shift-right: [w1994] -> _
    shift-left: w11 -> [w1998]
    shift-right: [w1993] -> _
    shift-left: w10 -> [w1997]
    shift-right: [w1991] -> _
    shift-left: w9 -> [w1992]
    shift-right: [w1988] -> _
    shift-left: w8 -> [w1989]
    shift-right: [w1987] -> _
    shift-left: w8 -> [w1990]
    shift-right: [w1980] -> _
    shift-left: w8 -> [w1986]
    shift-right: [w1979] -> _
    shift-left: w8 -> [w1985]
    shift-right: [w1978] -> _
    shift-left: w8 -> [w1984]
    shift-right: [w1977] -> _
    shift-left: w8 -> [w1983]
    shift-right: [w1976] -> _
    shift-left: w8 -> [w1982]
    shift-right: [w1975] -> _
    shift-left: w8 -> [w1981]
    shift-right: [w1974] -> _
    shift-left: w8 -> [w1968]
    shift-right: [w1973] -> _
    shift-left: w8 -> [w1967]
    shift-right: [w1972] -> _
    shift-left: w8 -> [w1966]
    shift-right: [w1971] -> _
    shift-left: w8 -> [w1965]
    shift-right: [w1970] -> _
    shift-left: w8 -> [w1964]
    shift-right: [w1969] -> _
    shift-left: w8 -> [w1963]
    shift-right: [w1954] -> _
    shift-left: w8 -> [w1957]
    shift-right: [w1953] -> _
    shift-left: w8 -> [w1956]
    shift-right: [w1952] -> _
    shift-left: w8 -> [w1955]
    stop <- w2002 stop-if-true
    n1811 = local read "Read UNO"() -> (w1961:string)
    n1812 = local read "Error  2"() -> (w2001:errorcluster)
    n1813 = String Length(string=w1961) -> (length=w1960:i32)
    n1814 = call <vilib>:"Trim Whitespace.vi"("string"=w1961) -> ("trimmed string"=w1962:string)  [unwired: 1 in]
    n1815 = Greater Or Equal?(x=w1960, y=23) -> (x >= y?=w1958:bool)
    n1816 = case shown="No Error" w2001 {
      tunnel: w2000 -> [w2048 w2144]
      tunnel: w1999 -> [w2047 w2143]
      tunnel: w1998 -> [w2046 w2142]
      tunnel: w1997 -> [w2045 w2141]
      tunnel: [w2044 w2144] -> w1996
      tunnel: [w2043 w2143] -> w1995
      tunnel: [w2042 w2142] -> w1994
      tunnel: [w2041 w2141] -> w1993
      tunnel: w1992 -> [w2040 w2140]
      tunnel: [w2039 w2140] -> w1991
      tunnel: w1989 -> [w2038 w2139]
      tunnel: w1990 -> [w2037 w2138]
      tunnel: [w2036 w2139] -> w1988
      tunnel: [w2035 w2138] -> w1987
      tunnel: w1986 -> [w2034 w2137]
      tunnel: w1985 -> [w2033 w2136]
      tunnel: w1984 -> [w2032 w2135]
      tunnel: w1983 -> [w2031 w2134]
      tunnel: w1982 -> [w2030 w2133]
      tunnel: w1981 -> [w2029 w2132]
      tunnel: [w2028 w2137] -> w1980
      tunnel: [w2027 w2136] -> w1979
      tunnel: [w2026 w2135] -> w1978
      tunnel: [w2025 w2134] -> w1977
      tunnel: [w2024 w2133] -> w1976
      tunnel: [w2023 w2132] -> w1975
      tunnel: w1968 -> [w2022 w2131]
      tunnel: [w2021 w2131] -> w1974
      tunnel: [w2020 w2127] -> w1973
      tunnel: [w2019 w2126] -> w1972
      tunnel: [w2018 w2130] -> w1971
      tunnel: [w2017 w2129] -> w1970
      tunnel: [w2016 w2128] -> w1969
      tunnel: w1967 -> [w2015 w2130]
      tunnel: w1966 -> [w2014 w2129]
      tunnel: w1965 -> [w2013 w2128]
      tunnel: w1964 -> [w2012 w2127]
      tunnel: w1963 -> [w2011 w2126]
      tunnel: w1962 -> [w2010 _]
      tunnel: w1958 -> [w2009 _]
      tunnel: w1957 -> [w2008 w2125]
      tunnel: w1956 -> [w2007 w2124]
      tunnel: w1955 -> [w2006 w2123]
      tunnel: [w2005 w2125] -> w1954
      tunnel: [w2004 w2124] -> w1953
      tunnel: [w2003 w2123] -> w1952
      frame No Error {
        n1817 = case shown="True" w2009 {
          tunnel: w2048 -> [w2064 w2116]
          tunnel: w2047 -> [w2063 w2115]
          tunnel: w2046 -> [w2062 w2114]
          tunnel: w2045 -> [w2061 w2113]
          tunnel: [w2064 w2112] -> w2044
          tunnel: [w2063 w2111] -> w2043
          tunnel: [w2062 w2110] -> w2042
          tunnel: [w2061 w2109] -> w2041
          tunnel: w2040 -> [w2060 w2107]
          tunnel: [w2060 w2106] -> w2039
          tunnel: w2038 -> [w2059 w2105]
          tunnel: w2037 -> [w2058 w2104]
          tunnel: [w2059 w2103] -> w2036
          tunnel: [w2058 w2102] -> w2035
          tunnel: w2034 -> [w2057 w2101]
          tunnel: w2033 -> [w2056 w2100]
          tunnel: w2032 -> [w2055 w2099]
          tunnel: w2031 -> [w2054 w2098]
          tunnel: w2030 -> [w2053 w2097]
          tunnel: w2029 -> [w2052 w2096]
          tunnel: [w2057 w2095] -> w2028
          tunnel: [w2056 w2094] -> w2027
          tunnel: [w2055 w2093] -> w2026
          tunnel: [w2054 w2092] -> w2025
          tunnel: [w2053 w2091] -> w2024
          tunnel: [w2052 w2090] -> w2023
          tunnel: w2022 -> [w2070 w2089]
          tunnel: [w2070 w2088] -> w2021
          tunnel: [w2067 w2087] -> w2020
          tunnel: [w2066 w2086] -> w2019
          tunnel: [w2069 w2085] -> w2018
          tunnel: [w2065 w2084] -> w2017
          tunnel: [w2068 w2083] -> w2016
          tunnel: w2015 -> [w2069 w2082]
          tunnel: w2014 -> [w2068 w2081]
          tunnel: w2013 -> [w2067 w2080]
          tunnel: w2012 -> [w2066 w2079]
          tunnel: w2011 -> [w2065 w2078]
          tunnel: w2010 -> [_ w2077]
          tunnel: w2008 -> [w2051 w2076]
          tunnel: w2007 -> [w2050 w2075]
          tunnel: w2006 -> [w2049 w2074]
          tunnel: [w2051 w2073] -> w2005
          tunnel: [w2050 w2072] -> w2004
          tunnel: [w2049 w2071] -> w2003
          frame False {
          }
          frame True {
            n1818 = Tick Count (ms)() -> (millisecond timer value=w2108:u32)
            n1819 = String To Byte Array(string=w2077) -> (unsigned byte array=w2121:u8[])
            n1820 = Array Size(array=w2121) -> (size(s)=w2120:i32)
            n1821 = formula code="// --- INTERNAL VARIABLE DECLARATIONS ---\nint i = 0;\nint k = 0;\nint start_idx = -1;\nint end_idx = -1;\nint phase = 0;\nint sign0 = 1;\nint sign1 = 1;\nint ch0_val = 0;   \nint ch1_val = 0;   \nfloat ch0_raw = 0.0;\nfloat ch1_raw = 0.0;\nfloat temp0 = 0.0;\nfloat temp1 = 0.0;\nfloat ch0_clean = 0.0;\nfloat ch1_clean = 0.0;\n\nint valid_samples = 0; // FIX: Track if we actually parsed new data this window\nfloat max_allowed_bits = 8388607.0; // FIX: Change this to match your ADC max value\n\n// Temporal intermediate variables for calculation smoothing\nfloat raw_p2p_v = 0.0;\nfloat raw_friction = 0.0;\nfloat raw_cof = 0.0;\n\n// Temporal intermediate variables for Piezo voltage translations\nfloat piezo_min_v = 0.0;\nfloat piezo_max_v = 0.0;\n\n// Initialize output variables to current shift register states right away\nout_LVDT_Min_V = in_LVDT_Min_V;\nout_LVDT_Max_V = in_LVDT_Max_V;\nout_LVDT_P2P_V = in_LVDT_P2P_V;\nout_Piezo_P2P = in_Piezo_P2P;\nout_Friction_N = in_Friction_N;\nout_COF = in_COF;\nwindow_ready = 0;\n\n// --- STEP 1: PARSE EVERY STRING IN THE BYTE ARRAY ---\nif (array_size > 2) {\n    for (i = 0; i < array_size - 1; i++) {\n        if (raw_bytes[i] == 42) { // '*' character detected\n            start_idx = i;\n        }\n        \n        // Match standard delimiter sequence \";&\" or end window character\n        if (raw_bytes[i] == 59 && raw_bytes[i+1] == 38 && start_idx != -1) { \n            end_idx = i;\n            ch0_val = 0;\n            ch1_val = 0;\n            sign0 = 1;\n            sign1 = 1;\n            phase = 0; \n\n            for (k = start_idx + 1; k < end_idx; k++) {\n                if (raw_bytes[k] == 45) { // '-' sign\n                    if (phase == 0) sign0 = -1;\n                    else sign1 = -1;\n                }\n                else if (raw_bytes[k] == 43) { // '+' sign\n                    if (phase == 0) sign0 = 1;\n                    else sign1 = 1;\n                }\n                else if (raw_bytes[k] == 59) { // ';' delimiter\n                    phase = 1; \n                }\n                else if (raw_bytes[k] >= 48 && raw_bytes[k] <= 57) { // Numeric ASCII digits\n                    if (phase == 0) {\n                        ch0_val = (ch0_val * 10) + (raw_bytes[k] - 48);\n                    } else {\n                        ch1_val = (ch1_val * 10) + (raw_bytes[k] - 48);\n                    }\n                }\n            }\n\n            // Implicit type conversion\n            ch0_raw = ch0_val * sign0 * 1.0;\n            ch1_raw = ch1_val * sign1 * 1.0;\n\n            // FIX: Sanity check / Hard-clamping to catch sudden massive ASCII noise spikes\n            if (ch0_raw > max_allowed_bits)  ch0_raw = max_allowed_bits;\n            if (ch0_raw < -max_allowed_bits) ch0_raw = -max_allowed_bits;\n            if (ch1_raw > max_allowed_bits)  ch1_raw = max_allowed_bits;\n            if (ch1_raw < -max_allowed_bits) ch1_raw = -max_allowed_bits;\n\n            // --- STEP 2: 3-SAMPLE MEDIAN FILTER ---\n            m0_2 = m0_1; m0_1 = m0_0; m0_0 = ch0_raw;\n            float s0_0 = m0_0; float s0_1 = m0_1; float s0_2 = m0_2;\n            if (s0_0 > s0_1) { temp0 = s0_0; s0_0 = s0_1; s0_1 = temp0; }\n            if (s0_1 > s0_2) { temp0 = s0_1; s0_1 = s0_2; s0_2 = temp0; }\n            if (s0_0 > s0_1) { temp0 = s0_0; s0_0 = s0_1; s0_1 = temp0; }\n            ch0_clean = s0_1;\n\n            m1_2 = m1_1; m1_1 = m1_0; m1_0 = ch1_raw;\n            float s1_0 = m1_0; float s1_1 = m1_1; float s1_2 = m1_2;\n            if (s1_0 > s1_1) { temp1 = s1_0; s1_0 = s1_1; s1_1 = temp1; }\n            if (s1_1 > s1_2) { temp1 = s1_1; s1_1 = s1_2; s1_2 = temp1; }\n            if (s1_0 > s1_1) { temp1 = s1_0; s1_0 = s1_1; s1_1 = temp1; }\n            ch1_clean = s1_1;\n\n            // --- STEP 3: EXPONENTIAL FILTER (STREAM LEVEL) ---\n            if (ch0_filt == 0.0) ch0_filt = ch0_clean;\n            if (ch1_filt == 0.0) ch1_filt = ch1_clean;\n\n            ch0_filt = ch0_filt + (ch0_clean - ch0_filt) * 0.125;\n            ch1_filt = ch1_filt + (ch1_clean - ch1_filt) * 0.125;\n\n            // --- STEP 4: MIN/MAX WINDOW CONTINUOUS ACCUMULATION ---\n            if (ch0_filt > max_ch0) max_ch0 = ch0_filt;\n            if (ch0_filt < min_ch0) min_ch0 = ch0_filt;\n            if (ch1_filt > max_ch1) max_ch1 = ch1_filt;\n            if (ch1_filt < min_ch1) min_ch1 = ch1_filt;\n\n            valid_samples++; // FIX: Successfully parsed and accumulated a clean point\n            start_idx = -1; \n        }\n    }\n}\n\n// --- STEP 5: WINDOW EVALUATION ENGINE ---\n// FIX: Condition updated to verify that valid samples exist for both channels\nif (((current_time_ms - start_time_ms) >= 50) && (valid_samples > 0) && (min_ch0 < 9000000.0) && (min_ch1 < 9000000.0)) {\n    window_ready = 1;\n\n    // Linear Bit-to-Voltage Transformations (LVDT - Channel 0)\n    out_LVDT_Min_V = (min_ch0 * VREF) / 8388607.0;\n    out_LVDT_Max_V = (max_ch0 * VREF) / 8388607.0;\n    raw_p2p_v = out_LVDT_Max_V - out_LVDT_Min_V;\n\n    // Linear Bit-to-Voltage Transformations (Piezo - Channel 1)\n    piezo_min_v = (min_ch1 * VREF) / 8388607.0;\n    piezo_max_v = (max_ch1 * VREF) / 8388607.0;\n    \n    // Assign Peak-to-Peak Voltage directly to output indicator (Matches Python logic)\n    out_Piezo_P2P = piezo_max_v - piezo_min_v;\n    \n    // Force scaling calculations using Voltage delta * Newtons/Volt Factor\n    raw_friction = out_Piezo_P2P * PIEZO_CAL_FACTOR ;\n    raw_cof = raw_friction / NORMAL_FORCE;\n\n    // --- STEP 6: OUTPUT METRIC SMOOTHING (Low-Pass Filter Alpha = 0.05) ---\n    // Seed initial historical metrics if first loop iteration\n    if (hist_LVDT_P2P == 0.0) hist_LVDT_P2P = raw_p2p_v;\n    if (hist_Friction == 0.0) hist_Friction = raw_friction;\n    if (hist_COF == 0.0)      hist_COF = raw_cof;\n\n    // Apply exponential output dampening\n    hist_LVDT_P2P = hist_LVDT_P2P + (raw_p2p_v - hist_LVDT_P2P) * 0.05;\n    hist_Friction = hist_Friction + (raw_friction - hist_Friction) * 0.05; // Note: Can drop to 0.02 for more aggressive damping\n    hist_COF      = hist_COF + (raw_cof - hist_COF) * 0.05;\n\n    // Direct smoothed parameters out to UI Indicators\n    out_LVDT_P2P_V = hist_LVDT_P2P;\n    out_Friction_N = hist_Friction;\n    out_COF        = hist_COF;\n\n    // Reset tracking targets to extreme boundaries safely\n    min_ch0 = 9999999.0;\n    max_ch0 = -9999999.0;\n    min_ch1 = 9999999.0;\n    max_ch1 = -9999999.0;\n\n    valid_samples = 0; // FIX: Reset counter for next time frame\n    start_time_ms = current_time_ms;\n}"("raw_bytes"=w2121, "array_size"=w2120, "VREF"="VREF", "PIEZO_CAL_FACTOR"="PIEZO_CAL_FACTOR", "NORMAL_FORCE"="NORMAL_FORCE", "min_ch0"=w2116, "max_ch0"=w2115, "min_ch1"=w2114, "max_ch1"=w2113, "current_time_ms"=w2108, "start_time_ms"=w2107, "ch0_filt"=w2105, "ch1_filt"=w2104, "m0_0"=w2101, "m0_1"=w2100, "m0_2"=w2099, "m1_0"=w2098, "m1_1"=w2097, "m1_2"=w2096, "in_LVDT_Min_V"=w2089, "in_LVDT_Max_V"=w2082, "in_LVDT_P2P_V"=w2081, "in_Piezo_P2P"=w2080, "in_Friction_N"=w2079, "in_COF"=w2078, "hist_LVDT_P2P"=w2076, "hist_Friction"=w2075, "hist_COF"=w2074) -> ("window_ready"=→"Valid_data":dbl, "out_LVDT_Min_V"=w2088:dbl, "out_LVDT_Max_V"=w2087:dbl, "out_LVDT_P2P_V"=w2086:dbl, "out_Piezo_P2P"=w2085:dbl, "out_Friction_N"=w2084:dbl, "out_COF"=w2083:dbl, "min_ch0"=w2112:dbl, "max_ch0"=w2111:dbl, "min_ch1"=w2110:dbl, "max_ch1"=w2109:dbl, "start_time_ms"=w2106:u32, "ch0_filt"=w2103:dbl, "ch1_filt"=w2102:dbl, "m0_0"=w2095:dbl, "m0_1"=w2094:dbl, "m0_2"=w2093:dbl, "m1_0"=w2092:dbl, "m1_1"=w2091:dbl, "m1_2"=w2090:dbl, "hist_LVDT_P2P"=w2073:dbl, "hist_Friction"=w2072:dbl, "hist_COF"=w2071:dbl)
            "LVDT MIN" <- w2088
            "LVDT MAX" <- w2087
            "LVDT Peak" <- w2086
            "pizo raw" <- w2085
            "cof" <- w2083
            "Frictioin Force Raw" <- w2084
          }
        }
      }
      frame Error {
      }
    }
    n1822 = local read "Quit"() -> (w2002:bool)
  }
  n1823 = disable-structure shown="Disabled" {
    disable-tunnel: errorcluster {"status"=TRUE, "code"=0, "source"="Init"} ("error IO") -> [w2147 _]
    disable-tunnel: [w2145 _] -> w50
    frame Disabled {
      n1824 = while {
        shift-right: [w2163] -> w2149
        shift-left: _ -> [w2154]
        shift-right: [w2162] -> w2148
        shift-left: w2147 -> [w2156]
        tunnel: [w2151] -> w2145
        tunnel: [w2161] -> _
        i -> [w2161]
        stop <- w2151 stop-if-true
        n1825 = local read "Port 1a"() -> (w2157:bool)
        n1826 = local read "Port 3"() -> (w2158:bool)
        n1827 = local read "Com Port 1"() -> (w2155:refnum<visa-resource-name>)
        n1828 = Or(x=w2158, y=w2157) -> (x .or. y?=w2160:bool)
        n1829 = Unbundle(w2156) -> ("status"=→"Port 3":bool)  [unwired: 2 out]
        n1830 = Not Equal?(x=w2155, y=w2154) -> (x != y?=w2152:bool)
        n1831 = case shown="True" w2160 {
          frame False {
            w2166 = TRUE ("Visible")
            n1832 = property on="Port 1a" class="Bool (strict)"("Visible"=w2166) -> ()  [unwired: 2 in, 2 out]
            n1833 = property on="Port 3" class="Bool (strict)"("Visible"=w2166) -> ()  [unwired: 2 in, 2 out]
          }
          frame True {
            w2167 = TRUE ("Visible")
            n1834 = property on="Port 1a" class="Bool (strict)"("Visible"=w2167) -> ()  [unwired: 2 in, 2 out]
            n1835 = property on="Port 3" class="Bool (strict)"("Visible"=w2167) -> ()  [unwired: 2 in, 2 out]
          }
        }
        n1836 = Wait (ms)(milliseconds to wait=u32 40) -> ()  [unwired: 1 out]
        n1837 = case shown="True" w2152 {
          tunnel: [w2164 errorcluster {"status"=TRUE, "code"=0, "source"="Init"} ("error out")] -> w2153
          tunnel: w2156 -> [w2164 _]
          frame False {
          }
          frame True {
          }
        }
        n1838 = case shown="Error" w2153 {
          selector: w2153 -> [w2174 w2192]
          tunnel: [w2177 w2196] -> w2163
          tunnel: [w2176 w2190] -> w2162
          tunnel: w2154 -> [w2175 w2194]
          frame No Error {
            n1839 = property class="Instr"(reference=w2175, error in=w2174) -> (reference out=w2172:refnum<visa-resource-name>, error out=w2173:errorcluster, "Serial Settings:Number of Bytes at Serial Port"=w2169:u32)
            n1840 = Greater?(x=w2169, y=u32 5) -> (0:w2168:bool)
            n1841 = Not(x=w2168) -> (.not. x?=→"Port 1a":bool)
            n1842 = while {
              tunnel: [w2185] -> w2176
              tunnel: [w2184] -> w2177
              tunnel: w2173 -> [w2183]
              tunnel: w2172 -> [w2182]
              stop <- TRUE stop-if-true
              n1843 = property class="Instr" props=["Serial Settings:Number of Bytes at Serial Port"](reference=w2182, error in=w2183) -> (reference out=w2187:refnum<visa-resource-name>, error out=w2186:errorcluster)  [unwired: 1 out]
              n1844 = VISA Read(VISA resource name=w2187, byte count=u32 50, error in (no error)=w2186) -> (VISA resource name out=w2184:refnum<visa-resource-name>, read buffer=w2179:string, error out=w2185:errorcluster)  [unwired: 1 out]
              n1845 = Wait (ms)(milliseconds to wait=u32 5) -> ()  [unwired: 1 out]
            }
          }
          frame Error {
            w2202 = u16 0 items=["None", "XON/XOFF", "RTS/CTS", "XON/XOFF & RTS/CTS", "DTR/DSR", "XON/XOFF & DTR/DSR"] ("flow control (0:none)  2")
            w2200 = u16 10 items=["1.0"=10, "1.5"=15, "2.0"=20] ("stop bits 2")
            w2198 = u16 0 items=["None", "Odd", "Even", "Mark", "Space"] ("parity 2")
            w2199 = u32 10000  # timeout (10sec)
            n1846 = VISA Close(VISA resource name=w2194, error in (no error)=w2192) -> (error out=w2195:errorcluster)
            n1847 = local write "Port 1a"(FALSE ("Port 1a")) -> ()
            n1848 = local read "Com Port 1"() -> (w2189:refnum<visa-resource-name>)
            n1849 = call <vilib>:"Clear Errors.vi"("error in (no error)"=w2195) -> ("error out"=w2193:errorcluster)  [unwired: 5 in, 1 out]
            n1850 = call-poly "VISA Configure Serial Port"("VISA resource name"=w2189, "timeout (10sec)"=w2199, "baud rate (9600)"=u32 250000 ("baud rate  2"), "data bits (8)"=u16 8 ("data bits  2"), "parity (0:none)"=w2198, "error in (no error)"=w2193, "stop bits (10: 1 bit)"=w2200, "flow control (0:none)"=w2202) -> ("VISA resource name out"=w2203:refnum<visa-resource-name>, "error out"=w2204:errorcluster)  [unwired: 6 in]
            n1851 = flat-sequence {
              tunnel: w2203 -> [w2206]
              tunnel: w2204 -> [w2205]
              tunnel: [w2206] -> w2196
              tunnel: [w2205] -> w2190
              frame #0 {
                n1852 = Wait (ms)(milliseconds to wait=u32 50) -> ()  [unwired: 1 out]
              }
            }
            "Residual Uno" <- ""
          }
        }
        n1853 = local read "Quit"() -> (w2151:bool)
        "Error Uno" <- w2156
      }
      n1854 = VISA Close(VISA resource name=w2149, error in (no error)=w2148) -> (error out=w2146:errorcluster)
      n1855 = call <vilib>:"Clear Errors.vi"("error in (no error)"=w2146) -> ()  [unwired: 5 in, 2 out]
    }
    frame Enabled {
    }
  }
  n1856 = while {
    stop <- w2217 stop-if-true
    # "V0OLTAGE TO STROKE (peice vise calibration)"
    n1857 = local read "LVDT MIN"() -> (w2209:dbl)
    n1858 = local read "LVDT Peak"() -> (w2208:dbl)
    n1859 = Wait (ms)(milliseconds to wait=u32 10) -> ()  [unwired: 1 out]
    n1860 = formula code="// Dynamic Parameterized Linear Interpolation Node\n// Inputs: vpp_val, voltages (Array), distances (Array)\n// Outputs: stroke\n\nint i = 0;\nint segments = 11; // 12 points make 11 interpolation segments\n\n// 1. Lower Boundary Clamp\nif (vpp_val <= voltages[0]) {\n    stroke = distances[0];\n}\n// 2. Upper Boundary Clamp\nelse if (vpp_val >= voltages[segments]) {\n    stroke = distances[segments];\n}\n// 3. Dynamic Segment Search Loop\nelse {\n    stroke = distances[0]; // Fallback baseline\n    for (i = 0; i < segments; i++) {\n        if (vpp_val >= voltages[i] && vpp_val <= voltages[i+1]) {\n            // Standard linear interpolation formula using array lookups\n            stroke = distances[i] + (vpp_val - voltages[i]) * (distances[i+1] - distances[i]) / (voltages[i+1] - voltages[i]);\n            break; // Segment found, safely exit the loop\n        }\n    }\n}"("vpp_val"=w2208, "voltages"="calibration values", "distances"="STROKE") -> ("stroke"=→"LVDT STROKE":dbl)
    n1861 = local read "Calibration Tare Value"() -> (w2213:dbl)
    n1862 = local read "Calibration Tare"() -> (w2211:bool)
    n1863 = Subtract(x=w2209, y=w2213) -> (x-y=→"LVDT STROKE  Calibration":dbl)
    n1864 = case shown="True" w2211 {
      selector: w2211 -> [_ w2219]
      tunnel: w2209 -> [_ w2220]
      frame False {
      }
      frame True {
        n1865 = Not(x=w2219) -> (.not. x?=w2218:bool)
        n1866 = local write "Calibration Tare"(w2218) -> ()
        "Calibration Tare Value" <- w2220
      }
    }
    n1867 = local read "Quit"() -> (w2217:bool)
  }
  n1868 = while {
    stop <- w2243 stop-if-true
    n1869 = local read "Due read"() -> (w2241:string)
    n1870 = call <vilib>:"High Resolution Polling Wait.vi"("seconds to wait"=0.02) -> ()  [unwired: 10 in, 1 out]
    n1871 = local read "Frictioin Force Raw"() -> (w2223:dbl)
    n1872 = Spreadsheet String To Array(delimiter (Tab)=";", format string="", spreadsheet string=w2241, array type (2D Dbl)=string[] []) -> (array=w2238:string[])
    n1873 = Fract/Exp String To Number(string=w2238) -> (number=w2237:dbl[])  [unwired: 3 in, 1 out]
    n1874 = call <vilib>:"Median Filter PtByPt.vi"("rank"=2, "x"=w2223) -> ("Filtered x"=→"Friction":dbl)  [unwired: 2 in, 1 out]
    n1875 = Index Array(array=w2237) -> (element #1=→"Sample Temperature 2":dbl, element #2=→"Target Sample Temperature":dbl, element #3=→"Current Duty Cycle":dbl, element #4=→"Ambient Temperature":dbl, element #5=→"Dac Status":dbl, element #6=→"Vpp":dbl, element #7=→"Active Error Code":dbl, element #8=→"Kp":dbl, element #9=→"Ki":dbl, element #10=→"Kd":dbl, element #11=→"SampleRaw":dbl, element #12=→"AmbRaw":dbl)  [unwired: 12 in]
    n1876 = local read "Quit"() -> (w2243:bool)
  }
  n1877 = while {
    shift-right: [w2257] -> w46
    shift-left: _ -> [w2249]
    shift-right: [w2244] -> w45
    shift-left: errorcluster {"status"=FALSE, "code"=0, "source"="Init"} ("error out") -> [w2251]
    tunnel: [w2246] -> w49
    tunnel: [w2256] -> _
    i -> [w2256]
    stop <- w2246 stop-if-true
    n1878 = local read "Com Port 2"() -> (w2250:refnum<visa-resource-name>)
    n1879 = local read "Port 2a"() -> (w2252:bool)
    n1880 = Unbundle(w2251) -> ("status"=→"Port 4":bool)  [unwired: 2 out]
    n1881 = call <vilib>:"High Resolution Polling Wait.vi"("seconds to wait"=0.02) -> ()  [unwired: 10 in, 1 out]
    n1882 = local read "Port 4"() -> (w2253:bool)
    n1883 = Not Equal?(x=w2250, y=w2249) -> (x != y?=w2248:bool)
    n1884 = Or(x=w2253, y=w2252) -> (x .or. y?=w2255:bool)
    n1885 = case shown="False" w2255 {
      frame False {
        w2260 = TRUE ("Visible")
        n1886 = property on="Port 2a" class="Bool (strict)"("Visible"=w2260) -> ()  [unwired: 2 in, 2 out]
        n1887 = property on="Port 4" class="Bool (strict)"("Visible"=w2260) -> ()  [unwired: 2 in, 2 out]
      }
      frame True {
        w2261 = TRUE ("Visible")
        n1888 = property on="Port 2a" class="Bool (strict)"("Visible"=w2261) -> ()  [unwired: 2 in, 2 out]
        n1889 = property on="Port 4" class="Bool (strict)"("Visible"=w2261) -> ()  [unwired: 2 in, 2 out]
      }
    }
    n1890 = case shown="True" w2248 {
      tunnel: [w2258 errorcluster {"status"=TRUE, "code"=0, "source"="Init"} ("error out")] -> w2247
      tunnel: w2251 -> [w2258 _]
      frame False {
      }
      frame True {
      }
    }
    n1891 = case shown="No Error" w2247 {
      selector: w2247 -> [w2274 w2305]
      tunnel: [w2267 w2310] -> w2257
      tunnel: [w2275 w2303] -> w2244
      tunnel: w2249 -> [w2276 w2308]
      frame No Error {
        n1892 = property class="Instr" props=["Serial Settings:Number of Bytes at Serial Port"](reference=w2276, error in=w2274) -> (reference out=w2268:refnum<visa-resource-name>, error out=w2273:errorcluster)  [unwired: 1 out]
        n1893 = while {
          tunnel: [w2284] -> w2269
          tunnel: [w2283] -> w2270
          tunnel: w2273 -> [w2282]
          tunnel: w2268 -> [w2281]
          tunnel: [w2280] -> _
          i -> [w2280]
          stop <- TRUE stop-if-true
          n1894 = property class="Instr" props=["Serial Settings:Number of Bytes at Serial Port"](reference=w2281, error in=w2282) -> (reference out=w2286:refnum<visa-resource-name>, error out=w2285:errorcluster)  [unwired: 1 out]
          n1895 = VISA Read(VISA resource name=w2286, byte count=u32 1000, error in (no error)=w2285) -> (VISA resource name out=w2283:refnum<visa-resource-name>, read buffer=→"Due read":string, error out=w2284:errorcluster)  [unwired: 1 out]
        }
        n1896 = local read "Due Write"() -> (w2266:string)
        n1897 = call <vilib>:"Trim Whitespace.vi"("string"=w2266) -> ("trimmed string"=w2265:string)  [unwired: 1 in]
        n1898 = Not Equal?(x=w2265, y="") -> (x != y?=w2271:bool)
        n1899 = VISA Flush I/O Buffer(VISA resource name=w2270) -> (VISA resource name out=w2263:refnum<visa-resource-name>, error out=→"error out 10":errorcluster)  [unwired: 2 in]
        n1900 = case shown="True" w2271 {
